vi "CANSendMotorSpeed.vi"(7 "Remote":bool=TRUE, 8 "error in (no error)":errorcluster, 9 "Motor Speed RPM":u16, 10 "UUT":refnum<vi>, 11 "Cluster in":refnum<vi>) -> (0 "error out":errorcluster caption="错误输出")   [LabVIEW 2017]
uses:
  PCAN_Driver/ControlCAN.llb/VCI_CAN_OBJ.ctl
  PCAN_Driver/ControlCAN.lvlib
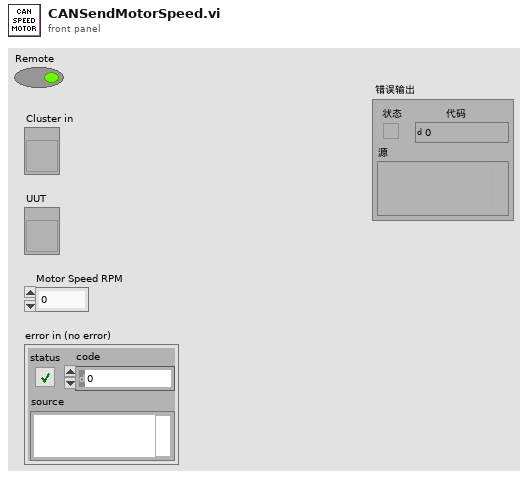
[diagram p1: front panel]
types:
  T1 = typedef "ControlCAN.lvlib/VCI_CAN_OBJ.ctl" = cluster{"ID":u32, "TimeStamp":u32, "TimeFlag":u8, "SendType":u8, "RemoteFlag":u8, "ExternFlag":u8, "DataLen":u8, "Data":u8[], "Reserved":u8[]}
  T2 = cluster{"ID":u32, "MSGTYPE":u8, "LEN":u8, "aDATA":u8[]}
  T3 = typedef "ControlCAN.lvlib/DevType.ctl" = u32
  T4 = typedef "ControlCAN.lvlib/CAN Channel.ctl" = u32
  T5 = typedef "ControlCAN.lvlib/VCI_INIT_CONFIG.ctl" = cluster{"AccCode":u32, "AccMask":u32, "InitFlag":T6, "Fliter":T7, "Timing0":u8, "Timing1":u8, "Mode":T8}
  T6 = typedef "ControlCAN.lvlib/InitFlag.ctl" = u32
  T7 = typedef "ControlCAN.lvlib/Fliter.ctl" = u8
  T8 = typedef "ControlCAN.lvlib/Mode.ctl" = u8
  T9 = cluster{"DevType":T3, "DevIndex":u32, "CanIndex":T4, "VCI_INIT_CONFIG":T5}
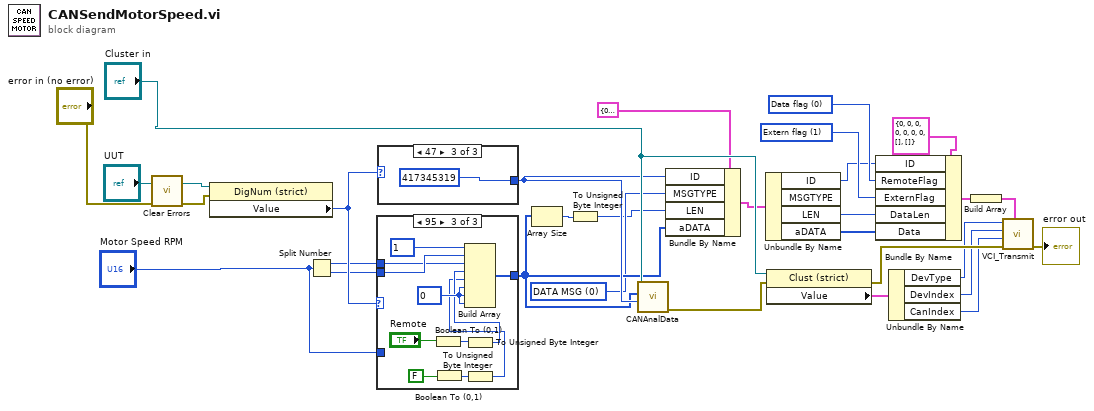
[diagram p0: block diagram]
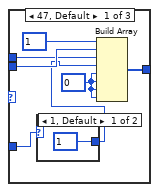
[diagram p2: hidden frame]
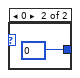
[diagram p3: hidden frame]
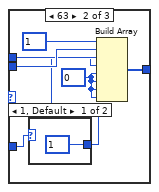
[diagram p4: hidden frame]
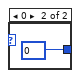
[diagram p5: hidden frame]
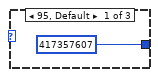
[diagram p6: hidden frame]
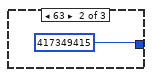
[diagram p7: hidden frame]
diagram:
  w18 = u8 0 items=["STATUS"=128, "EXTENDED"=2, "RTR"=1, "DATA MSG"=0] ("MSGTYPE")
  w13 = u8 1 items=["Standart flag", "Extern flag"] ("Format")
  w14 = u8 0 items=["Data flag", "Remote flag"] ("Type")
  n1 = call <vilib>:"Clear Errors.vi"("error in (no error)"="error in (no error)") -> ("error out"=w1:errorcluster)  [unwired: 5 in, 1 out]
  n2 = property on="Property Node" class="DigNum (strict)"(reference="UUT", error in=w1) -> ("Value"=w24:u8)  [unwired: 2 out]
  n3 = Split Number(x="Motor Speed RPM") -> (hi(x)=w22:u8, lo(x)=w21:u8)
  n4 = case shown="95" w24 {
    tunnel: [w37 w46 w59] -> w20
    tunnel: w21 -> [w36 w45 w58]
    tunnel: w22 -> [w35 w44 w57]
    tunnel: "Motor Speed RPM" -> [w32 w41 _]
    frame 47, Default {
      w34 = u8 0 ("element")
      n5 = case shown="1, Default" w32 {
        tunnel: [u8 1 ("element") u8 0 ("element")] -> w31
        frame 1, Default {
        }
        frame 0 {
        }
      }
      n6 = Build Array(u8 1 ("element"), w36, w35, w31, w34, w34, w34, w34) -> (w37:u8[])
    }
    frame 63 {
      w42 = u8 0 ("element")
      n7 = case shown="1, Default" w41 {
        tunnel: [u8 1 ("element") u8 0 ("element")] -> w40
        frame 1, Default {
        }
        frame 0 {
        }
      }
      n8 = Build Array(u8 1 ("element"), w45, w44, w40, w42, w42, w42, w42) -> (w46:u8[])
    }
    frame 95 {
      w55 = u8 0 ("element")
      n9 = Boolean To (0,1)(Boolean="Remote") -> (0, 1=w53:i16)
      n10 = Boolean To (0,1)(Boolean=FALSE ("Motor Over Temp 2")) -> (0, 1=w54:i16)
      n11 = To Unsigned Byte Integer(number=w53) -> (unsigned 8bit integer=w51:u8)
      n12 = To Unsigned Byte Integer(number=w54) -> (unsigned 8bit integer=w50:u8)
      n13 = Build Array(u8 1 ("element"), w58, w57, w51, w50, w55, w55, w55) -> (w59:u8[])
    }
  }
  n14 = case shown="47" w24 {
    tunnel: [u32 417357607 u32 417349415 u32 417345319] -> w23
    frame 95, Default {
    }
    frame 63 {
    }
    frame 47 {
    }
  }
  n15 = Array Size(array=w20) -> (size(s)=w15:i32)
  n16 = To Unsigned Byte Integer(number=w15) -> (unsigned 8bit integer=w17:u8)
  n17 = call "CANAnalData.vi"("ID"=w23, "Data"=w20, "Config"="Cluster in") -> ("error out"=w30:errorcluster)  [unwired: 4 in, 4 out]
  n18 = Bundle By Name(cluster=T2 {"ID"=0, "MSGTYPE"=0, "LEN"=0, "aDATA"=[]} ("MsgTX 2"), "ID"=w23, "MSGTYPE"=w18, "LEN"=w17, "aDATA"=w20) -> (w19:T2)
  n19 = Unbundle By Name(w19) -> ("ID"=w5:u32, "LEN"=w4:u8, "aDATA"=w3:u8[])  [unwired: 1 out]
  n20 = property class="Clust (strict)"(reference="Cluster in", error in=w30) -> (error out=w29:errorcluster, "Value"=w6:T9)  [unwired: 1 out]
  n21 = Bundle By Name(cluster=T1 {"ID"=0, "TimeStamp"=0, "TimeFlag"=0, "SendType"=0, "RemoteFlag"=0, "ExternFlag"=0, "DataLen"=0, "Data"=[], "Reserved"=[]} ("Send"), "ID"=w5, "RemoteFlag"=w14, "ExternFlag"=w13, "DataLen"=w4, "Data"=w3) -> (w8:T1)
  n22 = Unbundle By Name(w6) -> ("DevType"=w12:T3, "DevIndex"=w11:u32, "CanIndex"=w10:T4)
  n23 = Build Array(w8) -> (w9:T1[])
  n24 = call "VCI_Transmit.vi"("Buffer"=w9, "error in (no error)"=w29, "CANIndex"=w10, "DevIndex"=w11, "DevType"=w12) -> ("error out"=→"error out":errorcluster)  [unwired: 6 out]
